vi "decimalAdd.vi"(11 "inputString":string) -> (3 "resultString":string)   [LabVIEW 2018]
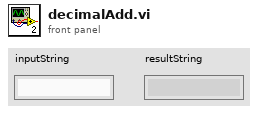
[diagram p1: front panel]
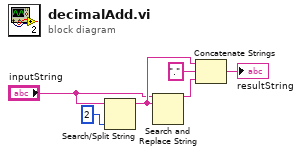
[diagram p0: block diagram]
diagram:
  n1 = Search/Split String(string="inputString", offset (0)=2) -> (substring before match=w3:string)  [unwired: 1 in, 2 out]
  n2 = Search and Replace String(input string="inputString", search string=w3) -> (result string=w4:string)  [unwired: 6 in, 3 out]
  n3 = Concatenate Strings(w3, "." ("string"), w4) -> (→"resultString":string)
